vi "SegmentDisplay.vi"(11 "Numeric":i64) -> (3 "new picture":picture)   [LabVIEW 2025]
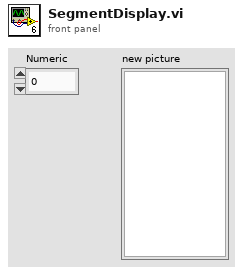
[diagram p1: front panel]
types:
  T1 = typedef "imagedata.ctl" = cluster{"image type":i32, "image depth":i32, "image":u8[], "mask":u8[], "colors":u32[], "Rectangle":cluster{"left":i16, "top":i16, "right":i16, "bottom":i16}}
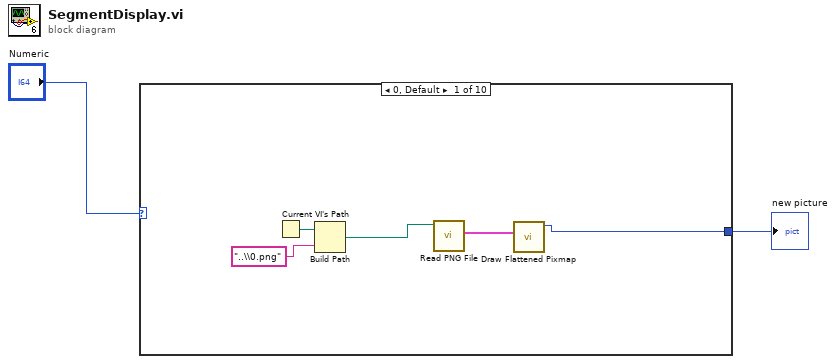
[diagram p0: block diagram]
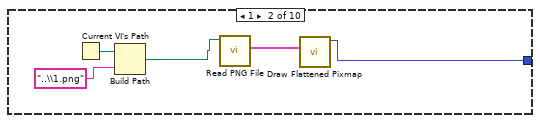
[diagram p2: hidden frame]
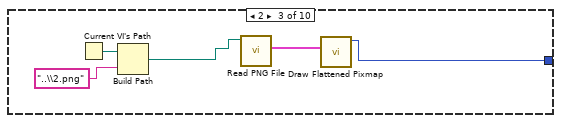
[diagram p3: hidden frame]
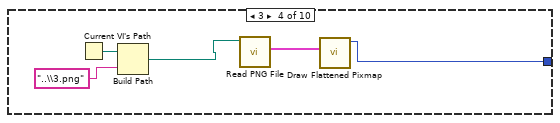
[diagram p4: hidden frame]
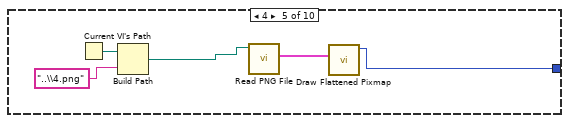
[diagram p5: hidden frame]
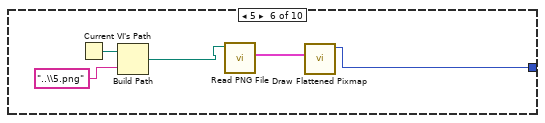
[diagram p6: hidden frame]
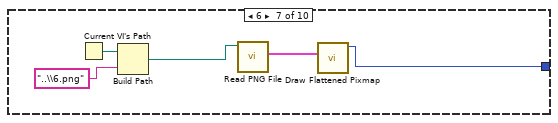
[diagram p7: hidden frame]
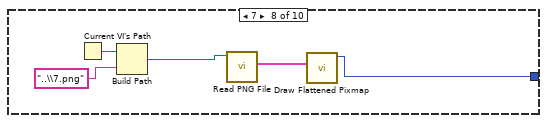
[diagram p8: hidden frame]
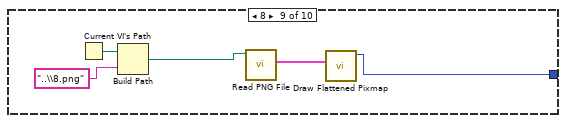
[diagram p9: hidden frame]
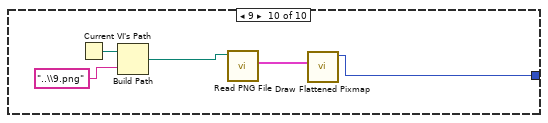
[diagram p10: hidden frame]
diagram:
  n1 = case shown="0, Default" "Numeric" {
    tunnel: [w3 w8 w13 w18 w23 w28 w33 w38 w43 w48] -> w2
    frame 0, Default {
      n2 = Current VI's Path() -> (path=w6:path)
      n3 = Build Path(base path=w6, name or relative path="..\\0.png") -> (appended path=w4:path)
      n4 = call <vilib>:"Read PNG File.vi"("path to PNG file"=w4) -> ("image data"=w7:T1)  [unwired: 8 in, 2 out]
      n5 = call <vilib>:"Draw Flattened Pixmap.vi"("image data"=w7) -> ("new picture"=w3:picture)  [unwired: 8 in]
    }
    frame 1 {
      n6 = Current VI's Path() -> (path=w11:path)
      n7 = Build Path(base path=w11, name or relative path="..\\1.png") -> (appended path=w9:path)
      n8 = call <vilib>:"Read PNG File.vi"("path to PNG file"=w9) -> ("image data"=w12:T1)  [unwired: 8 in, 2 out]
      n9 = call <vilib>:"Draw Flattened Pixmap.vi"("image data"=w12) -> ("new picture"=w8:picture)  [unwired: 8 in]
    }
    frame 2 {
      n10 = Current VI's Path() -> (path=w16:path)
      n11 = Build Path(base path=w16, name or relative path="..\\2.png") -> (appended path=w14:path)
      n12 = call <vilib>:"Read PNG File.vi"("path to PNG file"=w14) -> ("image data"=w17:T1)  [unwired: 8 in, 2 out]
      n13 = call <vilib>:"Draw Flattened Pixmap.vi"("image data"=w17) -> ("new picture"=w13:picture)  [unwired: 8 in]
    }
    frame 3 {
      n14 = Current VI's Path() -> (path=w21:path)
      n15 = Build Path(base path=w21, name or relative path="..\\3.png") -> (appended path=w19:path)
      n16 = call <vilib>:"Read PNG File.vi"("path to PNG file"=w19) -> ("image data"=w22:T1)  [unwired: 8 in, 2 out]
      n17 = call <vilib>:"Draw Flattened Pixmap.vi"("image data"=w22) -> ("new picture"=w18:picture)  [unwired: 8 in]
    }
    frame 4 {
      n18 = Current VI's Path() -> (path=w26:path)
      n19 = Build Path(base path=w26, name or relative path="..\\4.png") -> (appended path=w24:path)
      n20 = call <vilib>:"Read PNG File.vi"("path to PNG file"=w24) -> ("image data"=w27:T1)  [unwired: 8 in, 2 out]
      n21 = call <vilib>:"Draw Flattened Pixmap.vi"("image data"=w27) -> ("new picture"=w23:picture)  [unwired: 8 in]
    }
    frame 5 {
      n22 = Current VI's Path() -> (path=w31:path)
      n23 = Build Path(base path=w31, name or relative path="..\\5.png") -> (appended path=w29:path)
      n24 = call <vilib>:"Read PNG File.vi"("path to PNG file"=w29) -> ("image data"=w32:T1)  [unwired: 8 in, 2 out]
      n25 = call <vilib>:"Draw Flattened Pixmap.vi"("image data"=w32) -> ("new picture"=w28:picture)  [unwired: 8 in]
    }
    frame 6 {
      n26 = Current VI's Path() -> (path=w36:path)
      n27 = Build Path(base path=w36, name or relative path="..\\6.png") -> (appended path=w34:path)
      n28 = call <vilib>:"Read PNG File.vi"("path to PNG file"=w34) -> ("image data"=w37:T1)  [unwired: 8 in, 2 out]
      n29 = call <vilib>:"Draw Flattened Pixmap.vi"("image data"=w37) -> ("new picture"=w33:picture)  [unwired: 8 in]
    }
    frame 7 {
      n30 = Current VI's Path() -> (path=w41:path)
      n31 = Build Path(base path=w41, name or relative path="..\\7.png") -> (appended path=w39:path)
      n32 = call <vilib>:"Read PNG File.vi"("path to PNG file"=w39) -> ("image data"=w42:T1)  [unwired: 8 in, 2 out]
      n33 = call <vilib>:"Draw Flattened Pixmap.vi"("image data"=w42) -> ("new picture"=w38:picture)  [unwired: 8 in]
    }
    frame 8 {
      n34 = Current VI's Path() -> (path=w46:path)
      n35 = Build Path(base path=w46, name or relative path="..\\8.png") -> (appended path=w44:path)
      n36 = call <vilib>:"Read PNG File.vi"("path to PNG file"=w44) -> ("image data"=w47:T1)  [unwired: 8 in, 2 out]
      n37 = call <vilib>:"Draw Flattened Pixmap.vi"("image data"=w47) -> ("new picture"=w43:picture)  [unwired: 8 in]
    }
    frame 9 {
      n38 = Current VI's Path() -> (path=w51:path)
      n39 = Build Path(base path=w51, name or relative path="..\\9.png") -> (appended path=w50:path)
      n40 = call <vilib>:"Read PNG File.vi"("path to PNG file"=w50) -> ("image data"=w52:T1)  [unwired: 8 in, 2 out]
      n41 = call <vilib>:"Draw Flattened Pixmap.vi"("image data"=w52) -> ("new picture"=w48:picture)  [unwired: 8 in]
    }
  }
  "new picture" <- w2
